vi "cs-scanning.vi"() -> ()   [LabVIEW 2017]
uses:
  controls/boolean_info.ctl
  z-axis-params.ctl
  <vilib>/rvi/Emulation/niFpgaGetClockAttributes.vi
  <vilib>/rvi/Emulation/niFpgaSctlEmulationGetInTimedLoop.vi
  <vilib>/rvi/Emulation/niFpgaEmulationReportErrorSimple.vi
  <vilib>/rvi/Emulation/niFpgaProcessEmulError.vi
  <vilib>/rvi/eio/common/nirviEmuTemplateMethod_errors.vi
  <vilib>/rvi/Emulation/niFpgaEmulationIsFPGAContextNoSignature.vi
  <vilib>/rvi/DataTransferAndStorage/Container/Common/niFpgaContainerGetUniqueNameForEmu.vi
  <vilib>/rvi/Memory/Memory_Emulation/niFpgaMemoryEmulationCacheClearOnFirstRun.vi
  <vilib>/rvi/Memory/Memory_Emulation/nirvimemoryEmulationManagerCache_MakeExclusive.vi
  <vilib>/rvi/Memory/Memory_Emulation/niFpgaMemoryEmulationValidateCache.vi
  <vilib>/rvi/Memory/Memory_Emulation/nirvimemoryEmulationManagerCache_InsertValue.vi
  <vilib>/Utility/error.llb/Clear Errors.vi
  <vilib>/rvi/Memory/Memory_Emulation/nirvimemoryEmulationManagerCache_ReleaseExclusive.vi
  <vilib>/rvi/Memory/Memory_Emulation/nirvimemoryEmulationManagerCache_GetValue.vi
  <vilib>/rvi/Memory/Memory_Emulation/nirvimemoryEmulationManagerCache_SetValue.vi
  <vilib>/rvi/Emulation/niFpgaCriticalErrorInLSC.vi
  <vilib>/eio/EIONode/EIONode.xnode
  <vilib>/rvi/DataTransferAndStorage/Container/XNode/niFpgaContainer.xnode
  <vilib>/rvi/DataTransferAndStorage/Register/Emulation/niFpgaRegisterEmulation.vi
  FPGA-data-logging.lvlib
  libimaging-cs.lvlib
panel:
  in  "step_down_frac":fxp<+,8,1>
  out "state1-count":u64
  out "state5-count":u64
  out "state4-count":u64
  out "state3-count":u64
  out "state2-count":u64
  in  "collect all":bool
  in  "collect move":bool=TRUE
  out "iter":i32
  out "entity-index":i16
  out "All Done":bool
  in  "TsTicks":u32=1600
  in  "z-axis-params":T1={"TOL"=0.3, "ramp_rate"=0.0, "z_u_max"=5.0, "setpoint"=0.0, "Ki"=0.001, "Z_error_threshold"=0.0, "Z_settled_samples_threshold "=0, "z_UP"=0.0, "zup_N"=0} {"Z_error_threshold" format="%#_13g"; "ramp_rate" format="%#_13g"; "TOL" format="%#_13g"}
  out "number-settled-samples-Z":i16
  out "Current Case":i16
  out "boolean \nindicators":T2
  out "z-u(k)":sgl
  in  "ABORT":bool
  out "read fifo timeout":bool
  in  "numEntities":i16
  out "e(0) (threshhold init)":fxp<+/-,16,5>
  in  "init Z up":fxp<+/-,16,5>
  in  "trigger-0":bool
  out "number-settled-samples-y":i16
  out "number-settled-samples-x":i16
  in  "xy-error-threshold":sgl format="%#_13g"
  in  "settled-samples\nthreshold":i16
  in  "Ki-xy":sgl=0.001 format="%#_13g"
  in  "xy-bound":sgl
  in  "initial case":i16
  # "- If collect all = fasle and collect move = false,\nwe only collect measurement data.\n- If collect all = false, and collect move = true,\nwe collect measurement and move data.\n- If collect all = true, we collect everything."
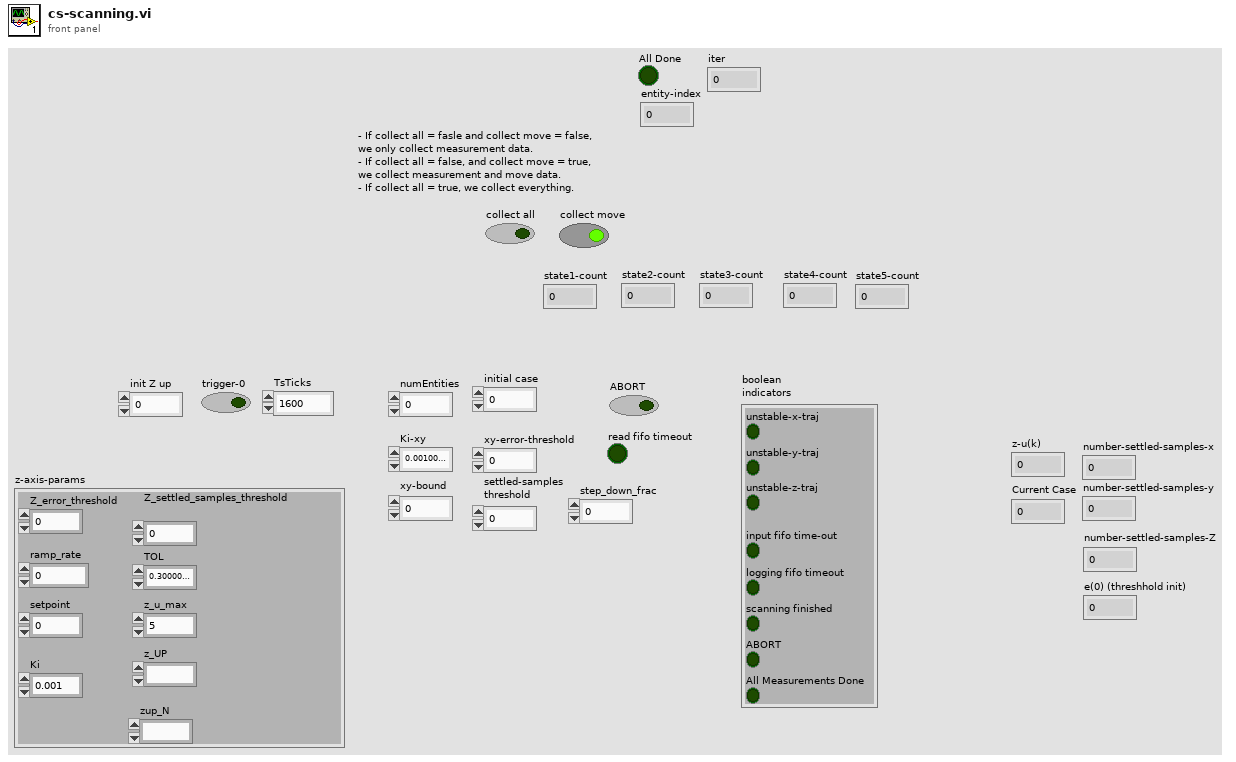
[diagram p1: front panel]
types:
  T1 = typedef "z-axis-params.ctl" = cluster{"TOL":sgl, "ramp_rate":sgl, "z_u_max":sgl, "setpoint":sgl, "Ki":sgl, "Z_error_threshold":sgl, "Z_settled_samples_threshold ":i16, "z_UP":fxp<+/-,16,5>, "zup_N":i16}
  T2 = typedef "boolean_info.ctl" = cluster{"unstable-z-traj":bool, "input fifo time-out":bool, "logging fifo timeout":bool, "scanning finished":bool, "unstable-x-traj":bool, "unstable-y-traj":bool, "ABORT":bool, "All Measurements Done":bool}
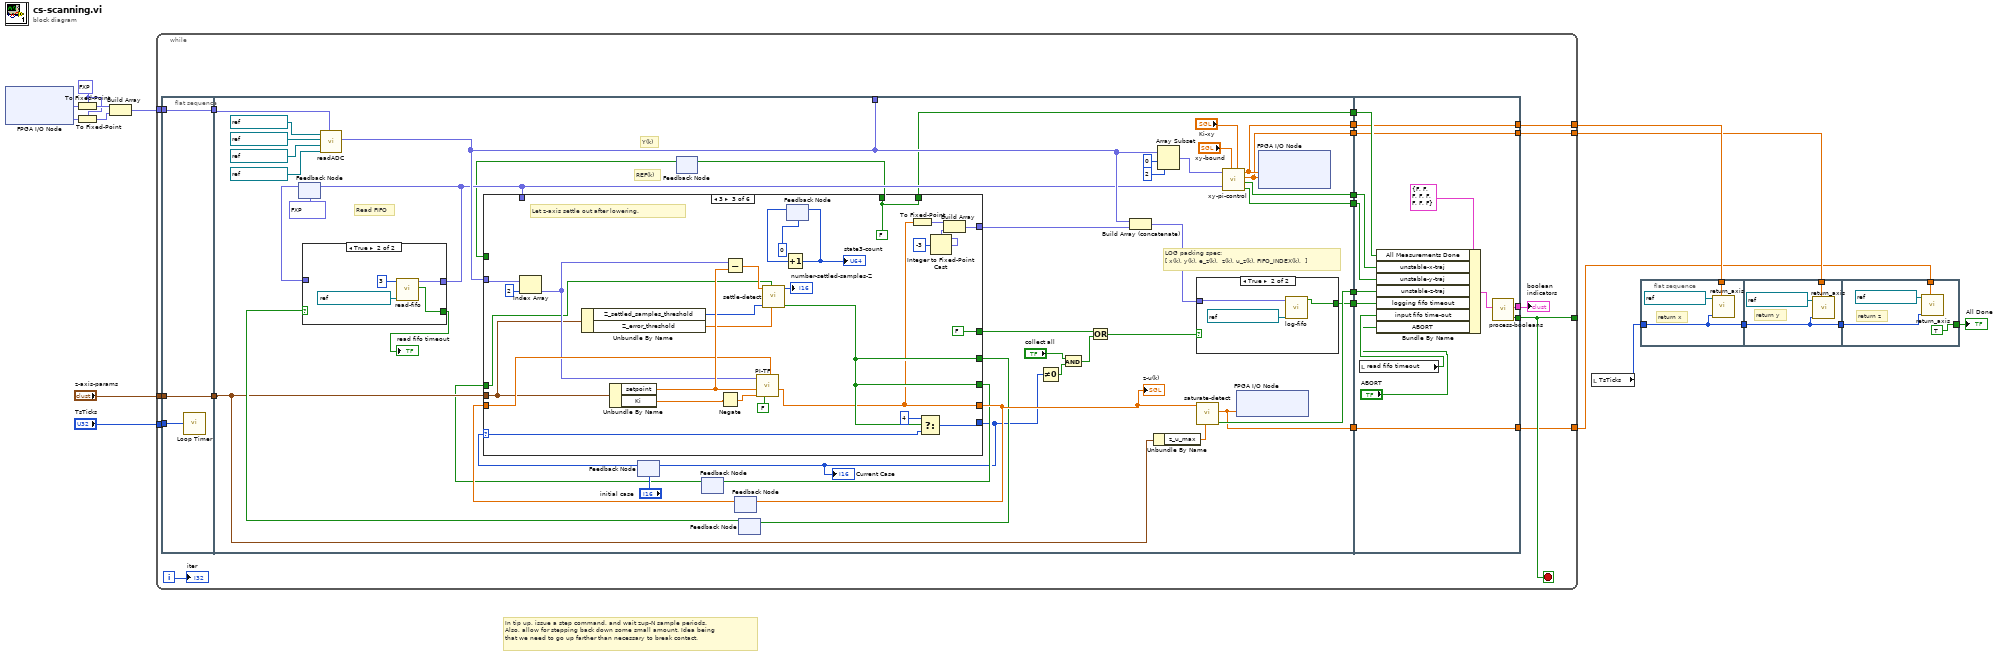
[diagram p0: block diagram]
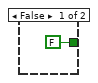
[diagram p2: hidden frame]
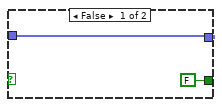
[diagram p3: hidden frame]
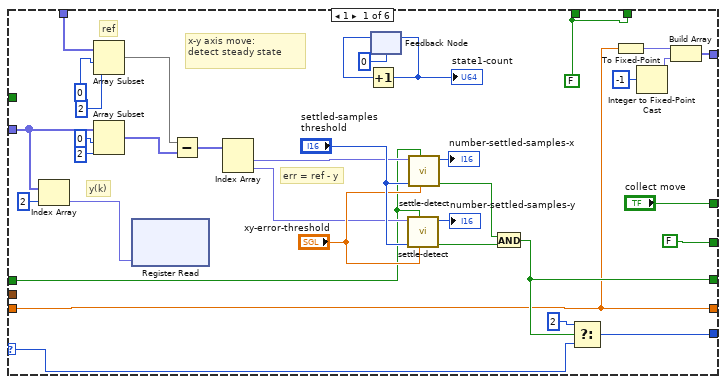
[diagram p4: hidden frame]
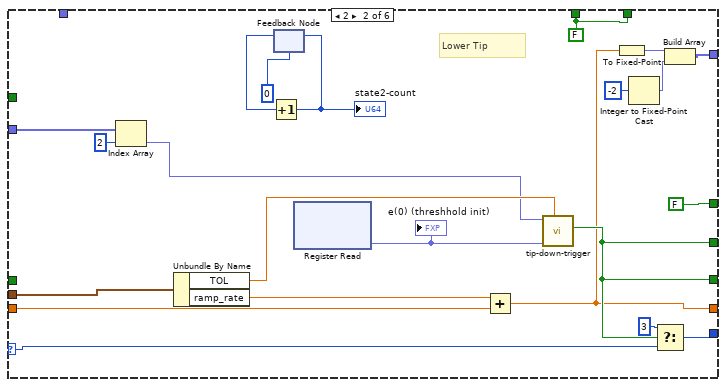
[diagram p5: hidden frame]
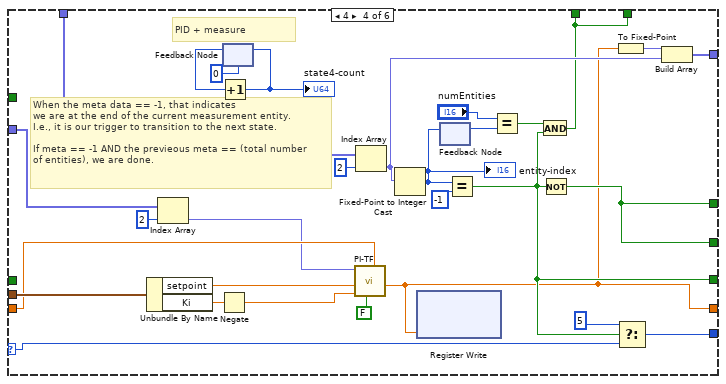
[diagram p6: hidden frame]
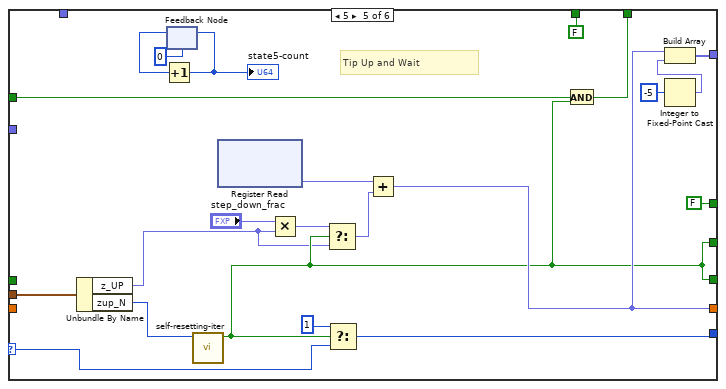
[diagram p7: hidden frame]
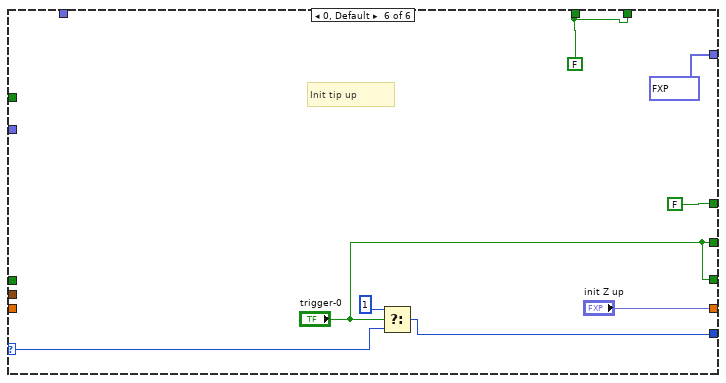
[diagram p8: hidden frame]
diagram:
  w10 = fxp<+/-,16,5> 0.0 ("fixed-point type")
  # "In tip up, issue a step command, and wait zup-N sample periods.\nAlso, allow for stepping back down some small amount. Idea being \nthat we need to go up farther than necessary to break contact."
  n1 = xnode "FPGA I/O Node"() -> ("Mod2/AI0"=w13:fxp<+/-,24,5>, "Mod2/AI1"=w11:fxp<+/-,24,5>)  [unwired: 2 in, 2 out]
  n2 = To Fixed-Point(fixed-point type=w10, number=w13) -> (fixed-point=w15:fxp<+/-,16,5>)
  n3 = To Fixed-Point(fixed-point type=w10, number=w11) -> (fixed-point=w12:fxp<+/-,16,5>)
  n4 = Build Array(w15, w12) -> (w14:fxp<+/-,16,5>[])
  n5 = while {
    tunnel: w14 -> [w27]
    tunnel: "z-axis-params" -> [w26]
    tunnel: "TsTicks" -> [w25]
    tunnel: [w23] -> _
    tunnel: [w21] -> w4
    tunnel: [w19] -> w3
    tunnel: [w17] -> w2
    i -> [w16]
    stop <- w23 stop-if-true
    n6 = flat-sequence {
      tunnel: w27 -> [w37]
      tunnel: [w37] -> w34
      tunnel: w25 -> [w35]
      tunnel: w26 -> [w36]
      tunnel: [w36] -> w33
      tunnel: w34 -> [w78]
      tunnel: w33 -> [w51]
      tunnel: [w64] -> w32
      tunnel: [w63] -> w31
      tunnel: [w62] -> w30
      tunnel: [w61] -> w29
      tunnel: [w47] -> w28
      tunnel: [w57] -> _
      tunnel: [w55] -> w22
      tunnel: [w54] -> w20
      tunnel: [w53] -> w18
      tunnel: w32 -> [w248]
      tunnel: w31 -> [w247]
      tunnel: w30 -> [w246]
      tunnel: w29 -> [w243]
      tunnel: w28 -> [w240]
      tunnel: [w239] -> w23
      tunnel: [w238] -> w24
      tunnel: w22 -> [w237]
      tunnel: [w237] -> w21
      tunnel: w20 -> [w236]
      tunnel: [w236] -> w19
      tunnel: [w235] -> w17
      tunnel: w18 -> [w235]
      frame #0 {
        n7 = call "Loop Timer"("Count(Ticks)"=w35) -> ()  [unwired: 1 out]
      }
      frame #1 {
        # "REF(k)"
        # "Y(k)"
        # "LOG packing spec:\n[ x(k), y(k), e_z(k),  z(k), u_z(k), FIFO_INDEX(k),  ]"
        # "Read FIFO"
        n8 = feedback #1(fxp<+/-,16,5>[] [0.0, 0.0, 0.0] ("unpacked-data")) -> (w69:fxp<+/-,16,5>[])
        n9 = call "readADC.vi"("x(0), y(0)"=w78, "z-height"=refnum<k21> "Mod2/AI3" ("y - ADC"), "z-err- ADC"=refnum<k21> "Mod2/AI2" ("y - ADC"), "y - ADC"=refnum<k21> "Mod2/AI1", "x - ADC"=refnum<k21> "Mod2/AI0") -> ("x_y_ze_z_k"=w57:fxp<+/-,17,6>[])  [unwired: 6 in]
        n10 = feedback #2("initial case") -> (w79:i16)
        n11 = feedback #3() -> (w48:bool)  [unwired: 1 in]
        n12 = feedback #4() -> (w45:bool)  [unwired: 1 in]
        n13 = feedback #5() -> (w67:sgl)  [unwired: 1 in]
        n14 = feedback #6() -> (w58:bool)  [unwired: 1 in]
        n15 = case shown="True" w58 {
          tunnel: w69 -> [w86 _]
          tunnel: [w86 w88] -> w52
          tunnel: [FALSE ("timout?") w87] -> w60
          frame False {
          }
          frame True {
            n16 = call "read-fifo.vi"("FIFO In"=refnum<k21> "Host_to_FPGA", "numChan"=3) -> ("timout?"=w87:bool, "unpacked-data"=w88:fxp<+/-,16,5>[])  [unwired: 8 in]
          }
        }
        "read fifo timeout" <- w60
        n17 = feedback-in #1(w52) -> ()
        n18 = case shown="3" w79 {
          selector: w79 -> [w117 w145 w163 w197 w224 w232]
          tunnel: ["collect move" FALSE FALSE ("trigger-0") w184 FALSE FALSE] -> w39
          tunnel: [w118 w140 w164 w198 w223 w234] -> w38
          tunnel: w57 -> [w112 w142 w168 w188 _ _]
          tunnel: [FALSE w135 w157 w184 w206 "trigger-0"] -> w59
          tunnel: [w91 w127 w149 w176 w210 "init Z up"] -> w66
          tunnel: w67 -> [w91 w138 w169 w194 _ _]
          tunnel: w51 -> [_ w144 w161 w199 w220 _]
          tunnel: [w104 w136 w158 w183 FALSE w229] -> w49
          tunnel: w52 -> [w105 _ _ w187 _ _]
          tunnel: w48 -> [_ _ _ _ w218 _]
          tunnel: [w104 w136 w158 w183 w217 w229] -> w47
          tunnel: w45 -> [w103 _ w148 _ _ _]
          tunnel: [w101 w135 w157 w182 w206 "trigger-0"] -> w46
          tunnel: [w99 w134 w156 w181 w216 fxp<+/-,16,5>[] [0.0, 0.0]] -> w44
          frame 1 {
            w104 = FALSE
            # "err = ref - y"
            # "y(k)"
            # "ref"
            # "x-y axis move: \ndetect steady state"
            n19 = Index Array(array=w112, index=2) -> (element=w109:fxp<+/-,17,6>)
            n20 = Array Subset(array=w105, index=0, length=2) -> (w111:fxp<+/-,16,5>[])
            n21 = Array Subset(array=w112, index=0, length=2) -> (w110:fxp<+/-,17,6>[])
            n22 = xnode ("Register Read")("Data"=w109) -> ()  [unwired: 1 in, 1 out]
            n23 = Subtract(x=w111, y=w110) -> (x-y=w100:fxp<+/-,18,7>[])
            n24 = Index Array(array=w100) -> (element #1=w107:fxp<+/-,18,7>, element #2=w106:fxp<+/-,18,7>)  [unwired: 2 in]
            n25 = feedback #7(u64 0) -> (w96:u64)
            n26 = Increment(x=w96) -> (x+1=w97:u64)
            "state1-count" <- w97
            n27 = feedback-in #7(w97) -> ()
            n28 = call "settle-detect.vi"("error-max"="xy-error-threshold", "reset"=w103, "settled-samples\nthreshold"="settled-samples\nthreshold", "err(k)"=w106) -> ("has-settled"=w125:bool, "number-settled-samples"=→"number-settled-samples-y":u16)  [unwired: 6 in]
            n29 = call "settle-detect.vi"("error-max"="xy-error-threshold", "reset"=w103, "settled-samples\nthreshold"="settled-samples\nthreshold", "err(k)"=w107) -> ("has-settled"=w124:bool, "number-settled-samples"=→"number-settled-samples-x":u16)  [unwired: 6 in]
            n30 = And(x=w124, y=w125) -> (x .and. y?=w101:bool)
            n31 = Select(t=i16 2, s=w101, f=w117) -> (s? t:f=w118:i16)
            n32 = To Fixed-Point(number=w91) -> (fixed-point=w92:fxp<+/-,16,5>)  [unwired: 1 in]
            n33 = Integer to Fixed-Point Cast(integer=i16 -1) -> (fixed-point=w93:fxp<+/-,16,5>)  [unwired: 1 in]
            n34 = Build Array(w92, w93) -> (w99:fxp<+/-,16,5>[])
          }
          frame 2 {
            w136 = FALSE
            # "Lower Tip"
            n35 = Index Array(array=w142, index=2) -> (element=w141:fxp<+/-,17,6>)
            n36 = Unbundle By Name(w144) -> ("TOL"=w147:sgl, "ramp_rate"=w146:sgl)
            n37 = feedback #8(u64 0) -> (w132:u64)
            n38 = Increment(x=w132) -> (x+1=w133:u64)
            "state2-count" <- w133
            n39 = feedback-in #8(w133) -> ()
            n40 = xnode ("Register Read")() -> ("Data"=w126:fxp<+/-,16,5>)  [unwired: 1 in, 1 out]
            "e(0) (threshhold init)" <- w126
            n41 = Add(x=w146, y=w138) -> (x+y=w127:sgl)
            n42 = call "tip-down-trigger.vi"("TOL"=w147, "Vo"=w126, "e(k)"=w141) -> ("trigger"=w135:bool)  [unwired: 8 in]
            n43 = To Fixed-Point(number=w127) -> (fixed-point=w128:fxp<+/-,16,5>)  [unwired: 1 in]
            n44 = Integer to Fixed-Point Cast(integer=i16 -2) -> (fixed-point=w129:fxp<+/-,16,5>)  [unwired: 1 in]
            n45 = Select(t=i16 3, s=w135, f=w145) -> (s? t:f=w140:i16)
            n46 = Build Array(w128, w129) -> (w134:fxp<+/-,16,5>[])
          }
          frame 3 {
            w158 = FALSE
            # "Let z-axis settle out after lowering."
            n47 = Index Array(array=w168, index=2) -> (element=w166:fxp<+/-,17,6>)
            n48 = Unbundle By Name(w161) -> ("Z_settled_samples_threshold"=w160:i16, "Z_error_threshold"=w159:sgl)
            n49 = Unbundle By Name(w161) -> ("setpoint"=w170:sgl, "Ki"=w173:sgl)
            n50 = Negate(x=w173) -> (-x=w174:sgl)
            n51 = Subtract(x=w166, y=w170) -> (x-y=w171:sgl)
            n52 = call "PI-TF.vi"("u(k-1)"=w169, "reset"=FALSE, "Ki"=w174, "setpoint"=w170, "y(k)"=w166) -> ("u(k)"=w149:sgl)  [unwired: 6 in]
            n53 = call "settle-detect.vi"("error-max"=w159, "reset"=w148, "settled-samples\nthreshold"=w160, "err(k)"=w171) -> ("has-settled"=w157:bool, "number-settled-samples"=→"number-settled-samples-Z":u16)  [unwired: 6 in]
            n54 = feedback #9(u64 0) -> (w154:u64)
            n55 = Increment(x=w154) -> (x+1=w155:u64)
            "state3-count" <- w155
            n56 = feedback-in #9(w155) -> ()
            n57 = To Fixed-Point(number=w149) -> (fixed-point=w150:fxp<+/-,16,5>)  [unwired: 1 in]
            n58 = Select(t=i16 4, s=w157, f=w163) -> (s? t:f=w164:i16)
            n59 = Integer to Fixed-Point Cast(integer=i16 -3) -> (fixed-point=w151:fxp<+/-,16,5>)  [unwired: 1 in]
            n60 = Build Array(w150, w151) -> (w156:fxp<+/-,16,5>[])
          }
          frame 4 {
            # "When the meta data == -1, that indicates\nwe are at the end of the current measurement entity.\nI.e., it is our trigger to transition to the next state.\n\nIf meta == -1 AND the previeous meta == (total number\nof entities), we are done."
            # "PID + measure"
            n61 = Unbundle By Name(w199) -> ("setpoint"=w202:sgl, "Ki"=w200:sgl)
            n62 = Index Array(array=w188, index=2) -> (element=w192:fxp<+/-,17,6>)
            n63 = Negate(x=w200) -> (-x=w201:sgl)
            n64 = feedback #10(u64 0) -> (w179:u64)
            n65 = Increment(x=w179) -> (x+1=w180:u64)
            "state4-count" <- w180
            n66 = feedback-in #10(w180) -> ()
            n67 = call "PI-TF.vi"("u(k-1)"=w194, "reset"=FALSE, "Ki"=w201, "setpoint"=w202, "y(k)"=w192) -> ("u(k)"=w176:sgl)  [unwired: 6 in]
            n68 = Index Array(array=w187, index=2) -> (element=w185:fxp<+/-,16,5>)
            n69 = Fixed-Point to Integer Cast(1:w185) -> (0:w186:i16)
            "entity-index" <- w186
            n70 = xnode ("Register Write")("Data"=w176) -> ()  [unwired: 1 in, 1 out]
            n71 = feedback #11() -> (w189:i16)  [unwired: 1 in]
            n72 = feedback-in #11(w186) -> ()
            n73 = Equal?(x=w186, y=i16 -1) -> (x = y?=w182:bool)
            n74 = Equal?(x="numEntities", y=w189) -> (x = y?=w190:bool)
            n75 = And(x=w190, y=w182) -> (x .and. y?=w183:bool)
            n76 = Not(x=w182) -> (.not. x?=w184:bool)
            n77 = To Fixed-Point(number=w176) -> (fixed-point=w177:fxp<+/-,16,5>)  [unwired: 1 in]
            n78 = Select(t=i16 5, s=w182, f=w197) -> (s? t:f=w198:i16)
            n79 = Build Array(w177, w185) -> (w181:fxp<+/-,16,5>[])
          }
          frame 5 {
            # "Tip Up and Wait"
            n80 = Unbundle By Name(w220) -> ("z_UP"=w205:fxp<+/-,16,5>, "zup_N"=w219:i16)
            n81 = feedback #12(u64 0) -> (w214:u64)
            n82 = Increment(x=w214) -> (x+1=w215:u64)
            "state5-count" <- w215
            n83 = feedback-in #12(w215) -> ()
            n84 = call "self-resetting-iter.vi"("N"=w219) -> ("Boolean"=w206:bool)  [unwired: 9 in, 1 out]
            n85 = xnode ("Register Read")() -> ("Data"=w221:fxp<+/-,16,5>)  [unwired: 1 in, 1 out]
            n86 = Multiply(x="step_down_frac", y=w205) -> (x*y=w209:fxp<+/-,24,6>)
            n87 = Select(t=w209, s=w206, f=w205) -> (s? t:f=w207:fxp<+/-,24,6>)
            n88 = Select(t=i16 1, s=w206, f=w224) -> (s? t:f=w223:i16)
            n89 = Add(x=w221, y=w207) -> (x+y=w210:fxp<+/-,25,7>)
            n90 = And(x=w218, y=w206) -> (x .and. y?=w217:bool)
            n91 = Integer to Fixed-Point Cast(integer=i16 -5) -> (fixed-point=w211:fxp<+/-,16,5>)  [unwired: 1 in]
            n92 = Build Array(w210, w211) -> (w216:fxp<+/-,25,7>[])
          }
          frame 0, Default {
            w229 = FALSE
            # "Init tip up"
            n93 = Select(t=i16 1, s="trigger-0", f=w232) -> (s? t:f=w234:i16)
          }
        }
        "z-u(k)" <- w66
        "Current Case" <- w38
        n94 = feedback-in #2(w38) -> ()
        n95 = feedback-in #3(w49) -> ()
        n96 = feedback-in #4(w46) -> ()
        n97 = feedback-in #5(w66) -> ()
        n98 = feedback-in #6(w59) -> ()
        n99 = Not Equal To 0?(x=w38) -> (x != 0?=w42:bool)
        n100 = And(x="collect all", y=w42) -> (x .and. y?=w40:bool)
        n101 = Or(x=w39, y=w40) -> (x .or. y?=w43:bool)
        n102 = Build Array (concatenate)(w57, w44) -> (w65:fxp<+/-,25,7>[])
        n103 = Unbundle By Name(w51) -> ("z_u_max"=w50:sgl)
        n104 = Array Subset(array=w57, index=0, length=2) -> (w68:fxp<+/-,17,6>[])
        n105 = case shown="True" w43 {
          tunnel: w65 -> [_ w83]
          tunnel: [FALSE ("logging-timeout?") w82] -> w61
          frame False {
          }
          frame True {
            n106 = call "log-fifo.vi"("FIFO In"=refnum<k21> "fpga-to-host2", "input-data"=w83) -> ("logging-timeout?"=w82:bool)  [unwired: 9 in]
          }
        }
        n107 = call "saturate-detect.vi"("bound"=w50, "x"=w66) -> ("saturated"=w62:bool, "sat(x)"=w53:sgl)  [unwired: 8 in]
        n108 = call "xy-pi-control.vi"("Ki-xy"="Ki-xy", "xy-umax"="xy-bound", "xy-ref"=w52, "x_k-y_k"=w68) -> ("u_y saturated"=w63:bool, "u_x saturated"=w64:bool, "sat(u_y)"=w54:sgl, "sat(u_x)"=w55:sgl)  [unwired: 4 in]
        n109 = xnode "FPGA I/O Node"("Mod1/AO2"=w53) -> ()  [unwired: 1 in, 1 out]
        n110 = xnode "FPGA I/O Node"("Mod1/AO0"=w55, "Mod1/AO1"=w54) -> ()  [unwired: 2 in, 2 out]
      }
      frame #2 {
        n111 = local read "read fifo timeout"() -> (w242:bool)
        n112 = Bundle By Name(cluster=T2 {"unstable-z-traj"=FALSE, "input fifo time-out"=FALSE, "logging fifo timeout"=FALSE, "scanning finished"=FALSE, "unstable-x-traj"=FALSE, "unstable-y-traj"=FALSE, "ABORT"=FALSE, "All Measurements Done"=FALSE} ("boolean errors"), "All Measurements Done"=w240, "unstable-x-traj"=w248, "unstable-y-traj"=w247, "unstable-z-traj"=w246, "logging fifo timeout"=w243, "input fifo time-out"=w242, "ABORT"="ABORT") -> (w244:T2)
        n113 = call "process-booleans.vi"("boolean indicators 2"=w244) -> ("scaning finished"=w239:bool, "boolean indicators"=w238:T2)  [unwired: 9 in]
      }
    }
    "boolean \nindicators" <- w24
    "iter" <- w16
  }
  n114 = local read "TsTicks"() -> (w5:u32)
  n115 = flat-sequence {
    tunnel: w5 -> [w250]
    tunnel: w4 -> [w251]
    tunnel: [w250] -> w7
    tunnel: w3 -> [w254]
    tunnel: w7 -> [w252]
    tunnel: [w252] -> w6
    tunnel: w2 -> [w258]
    tunnel: w6 -> [w256]
    tunnel: [TRUE] -> w1
    frame #0 {
      # "return x"
      n116 = call "return_axis.vi"("u(0)"=w251, "TsTicks"=w250, "FPGA I/O In"=refnum<k21> "Mod1/AO0") -> ()  [unwired: 9 in]
    }
    frame #1 {
      # "return y"
      n117 = call "return_axis.vi"("u(0)"=w254, "TsTicks"=w252, "FPGA I/O In"=refnum<k21> "Mod1/AO1") -> ()  [unwired: 9 in]
    }
    frame #2 {
      # "return z"
      n118 = call "return_axis.vi"("u(0)"=w258, "TsTicks"=w256, "FPGA I/O In"=refnum<k21> "Mod1/AO2") -> ()  [unwired: 9 in]
    }
  }
  "All Done" <- w1
